vi "Periodic Tasks.vi"(8 "error in":errorcluster) -> ()   [LabVIEW 2017]
doc: "This VI runs in parallel to other tasks. It can contain as many user-defined periodic loops as you need. These can carry out PID or other sorts of timed response."
uses:
  <vilib>/Rock Robotics/WPI/Utilities/WPI_GetSetVariantRefNum.vi
  <vilib>/Rock Robotics/WPI/ThirdParty/Sensors/ADIS16448 IMU/ADIS16448_IMU.lvlib
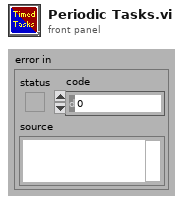
[diagram p1: front panel]
types:
  T1 = typedef "ADIS16448_IMU.lvlib/ADI_IMU_ADIS16448_IMUDevRef.ctl" = cluster{"DevStatus":errorcluster, "Handle":i32, "SPI Bus":T2, "Device Found":bool, "Device Ready":bool, "Yaw Axis":enum16{"X", "Y", "Z"}, "AHRS Algorithm":enum16{"Complementary", "Madgwick"}, "Serial":u16, "Lot ID 2":u16, "Lot ID 1":u16, "Bytes Per Sample":u16, "Calibrate On Open?":bool}
  T2 = typedef "spi_bus.ctl" = enum16{"SPI On-Board, CS0", "SPI On-Board, CS1", "SPI On-Board, CS2", "SPI On-Board, CS3", "SPI MXP", "Invalid"}
  T3 = typedef "WPI_JoystickDevRef.ctl" = cluster{"Device":T4}
  T4 = typedef "WPI_JoystickDeviceEnum.ctl" = enum16{"USB 0", "USB 1", "USB 2", "USB 3", "USB 4", "USB 5"}
  T5 = typedef "WPI_RobotDriveDevRef.ctl" = cluster{"DevStatus":errorcluster, "Motors[]":T6[], "Square Inputs":bool, "Max Output":dbl}
  T6 = typedef "WPI_MotorControlDeviceRef.ctl" = cluster{"DeviceStatus":errorcluster, "Type":T7, "PWM":cluster{"PWM Channel":T8, "DeadBand":T9}, "CAN":cluster{"Device Number":u8, "SetOutput VI Ref":variant, "GetOutput VI Ref":variant, "Enable VI Ref":variant, "Disable VI Ref":variant, "Data":variant}, "Invert":bool, "DIO PWM":cluster{"PWM \"Enable\" Channel":T8, "DIOChannel":T10, "PWM Rate":dbl}}
  T7 = typedef "WPI_MotorControlType.ctl" = enum16{"PWM", "CAN", "DIO PWM"}
  T8 = typedef "FPGA_DIOPWMChannel.ctl" = enum8{"PWM 0", "PWM 1", "PWM 2", "PWM 3", "PWM 4", "PWM 5", "PWM 6", "PWM 7", "PWM 8", "PWM 9", "PWM MXP 0", "PWM MXP 1", "PWM MXP 2", "PWM MXP 3", "PWM MXP 4", "PWM MXP 5", "PWM MXP 6", "PWM MXP 7", "PWM MXP 8", "PWM MXP 9", "Invalid"}
  T9 = typedef "WPI_PWMDeadband.ctl" = cluster{"Name":string, "maxPositivePwm":i32, "minPositivePwm":i32, "centerPwm":i32, "maxNegativePwm":i32, "minNegativePwm":i32, "angularRange":u16}
  T10 = typedef "FPGA_DIOChannel.ctl" = enum8{"DIO 0", "DIO 1", "DIO 2", "DIO 3", "DIO 4", "DIO 5", "DIO 6", "DIO 7", "DIO 8", "DIO 9", "DIO MXP 0", "DIO MXP 1", "DIO MXP 2", "DIO MXP 3", "DIO MXP 4", "DIO MXP 5", "DIO MXP 6", "DIO MXP 7", "DIO MXP 8", "DIO MXP 9", "DIO MXP 10", "DIO MXP 11", "DIO MXP 12", "DIO MXP 13", "DIO MXP 14", "DIO MXP 15", "SPI Port CS1", "SPI Port CS2", "SPI Port CS3", "SPI Port MISO", "SPI Port MOSI", "Invalid"}
  T11 = cluster{"JoystickDevRef":T3, "RobotDriveDevRef":T5}
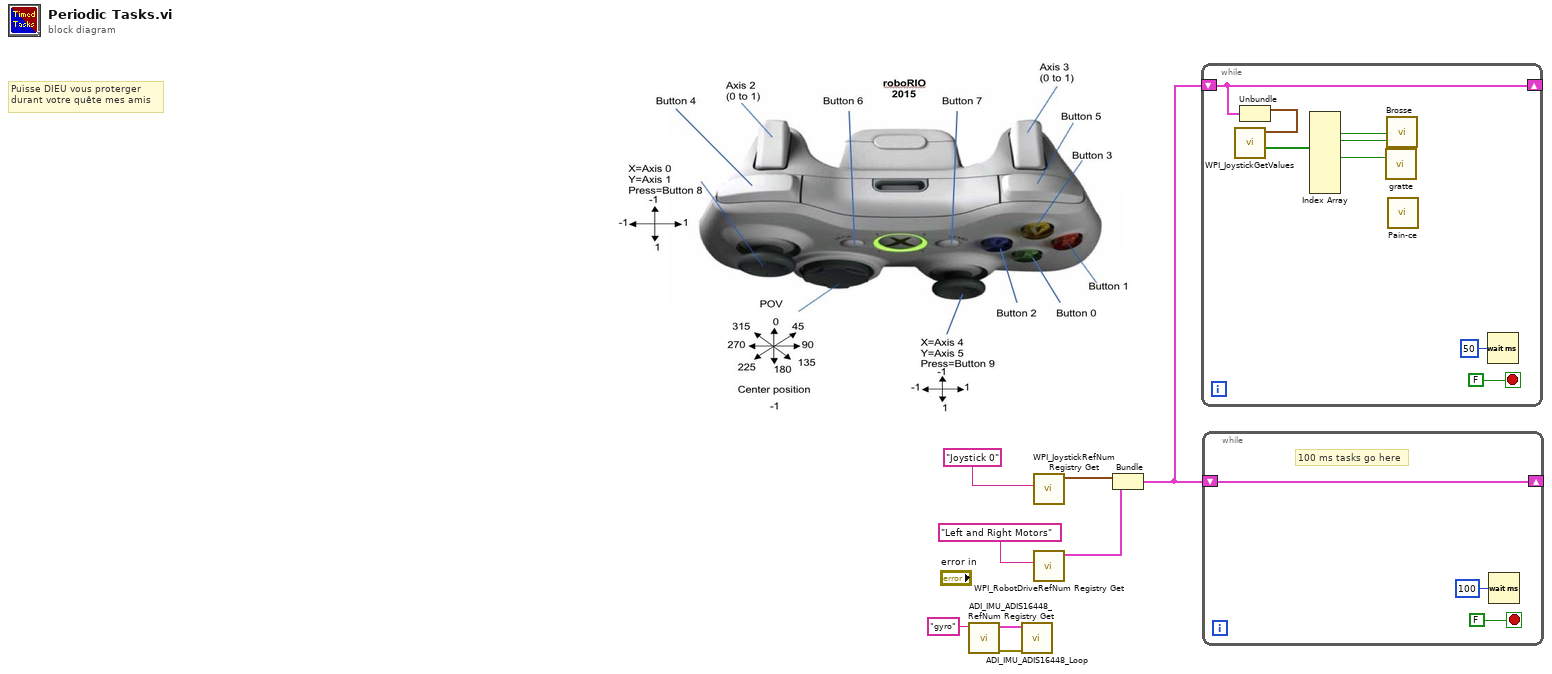
[diagram p0: block diagram]
diagram:
  # "Puisse DIEU vous proterger \ndurant votre quête mes amis"
  n1 = call <vilib>:"ADI_IMU_ADIS16448_RefNum Registry Get.vi"("refnum name"="gyro") -> ("error out"=w3:errorcluster, "ADI IMU DevRef"=w2:T1)  [unwired: 9 in]
  n2 = call <vilib>:"ADI_IMU_ADIS16448_Loop.vi"("error in"=w3, "ADI IMU DevRef"=w2) -> ()  [unwired: 9 in, 1 out]
  n3 = call <vilib>:"WPI_JoystickRefNum Registry Get.vi"("refnum name"="Joystick 0") -> ("JoystickDevRef"=w6:T3)  [unwired: 1 in, 9 out]
  n4 = call <vilib>:"WPI_RobotDriveRefNum Registry Get.vi"("refnum name"="Left and Right Motors") -> ("RobotDriveDevRef"=w5:T5)  [unwired: 1 in, 9 out]
  n5 = Bundle("JoystickDevRef"=w6, "RobotDriveDevRef"=w5) -> (w4:T11)  [unwired: 1 out]
  n6 = while {
    shift-right: [w11] -> _
    shift-left: w4 -> [w11]
    stop <- FALSE stop-if-true
    n7 = Unbundle(w11) -> ("JoystickDevRef"=w14:T3)  [unwired: 1 out]
    n8 = call <vilib>:"WPI_JoystickGetValues.vi"("JoystickDevRef"=w14) -> ("Buttons"=w13:bool[])  [unwired: 6 in, 4 out]
    n9 = Index Array(array=w13) -> (element #1=w10:bool, element #2=w9:bool, element #4=w12:bool)  [unwired: 8 in, 5 out]
    n10 = call "gratte.vi"("bouton gratte"=w12) -> ()
    n11 = call "Brosse.vi"("lift brosse"=w9, "brosse"=w10) -> ()
    n12 = call "Pain-ce.vi"() -> ()  [unwired: 2 in]
    n13 = Wait (ms)(milliseconds to wait=u32 50) -> ()  [unwired: 1 out]
  }
  n14 = while {
    shift-right: [w17] -> _
    shift-left: w4 -> [w17]
    stop <- FALSE stop-if-true
    # "100 ms tasks go here"
    n15 = Wait (ms)(milliseconds to wait=u32 100) -> ()  [unwired: 1 out]
  }
